vi "main.vi"() -> ()   [LabVIEW 2023] (continued)
8        17\t1F\t08\t60\tB1\t1F\t08\t55\r\n      2944  0CF102A7   00000004    8        30\t75\tE0\t2E\t80\tFF\tFF\tFD\r\n      2943  0C3C4D4A   00000004    8        BE\tFF\tFF\t7F\t18\tFF\tFF\t55\r\n      2943  0CF101A7   00000004    8        68\t00\t97\tCC\t00\t16\t39\tAD\r\n      2942  18F120F0   00000004    8        2B\t75\t60\tB1\tB0\t01\tFF\tFF\r\n      2941  18F11FF0   00000004    8        FF\t3F\t90\t68\t88\t1B\t10\t5C\r\n      2932  1FFFFFFF   00000004    8        00\t00\tFF\tFF\tFF\tFF\tFF\tFF\r\n      2923  0CF102A7   00000004    8        30\t75\tE0\t2E\t80\tFF\tFF\tFD\r\n      2923  0CF101A7   00000004    8        68\t00\t97\tCC\t00\t16\t39\tAC\r\n      2922  1FFFFFFF   00000004    8        00\t20\tFF\tFF\tFF\tFF\tFF\tFF\r\n      2945  18F106A7   00000004    8        00\tF7\tFF\tFF\tFF\tFF\tFF\tAB\r\n      2945  0CF104A7   00000004    8        F0\t60\t22\tFC\tFF\tFF\tFF\t55\r\n      2944  0CF103A7   00000004    8        17\t1F\t08\t60\tB1\t1F\t08\t55\r\n      2944  0CF102A7   00000004    8        30\t75\tE0\t2E\t80\tFF\tFF\tFD\r\n      2943  0C3C4D4A   00000004    8        BE\tFF\tFF\t7F\t18\tFF\tFF\t55\r\n      2943  0CF101A7   00000004    8        68\t00\t97\tCC\t00\t16\t39\tAD\r\n      2942  18F120F0   00000004    8        2B\t75\t60\tB1\tB0\t01\tFF\tFF\r\n      2941  18F11FF0   00000004    8        FF\t3F\t90\t68\t88\t1B\t10\t5C\r\n      2932  1FFFFFFF   00000004    8        00\t00\tFF\tFF\tFF\tFF\tFF\tFF\r\n      2923  0CF102A7   00000004    8        30\t75\tE0\t2E\t80\tFF\tFF\tFD\r\n      2923  0CF101A7   00000004    8        68\t00\t97\tCC\t00\t16\t39\tAC\r\n      2946  18F121F0   00000004    8        09\t19\t00\t00\tFF\tFF\tB0\t01\r\n      2945  18F106A7   00000004    8        00\tF7\tFF\tFF\tFF\tFF\tFF\tAB\r\n      2945  0CF104A7   00000004    8        F0\t60\t22\tFC\tFF\tFF\tFF\t55\r\n      2944  0CF103A7   00000004    8        17\t1F\t08\t60\tB1\t1F\t08\t55\r\n      2944  0CF102A7   00000004    8        30\t75\tE0\t2E\t80\tFF\tFF\tFD\r\n      2943  0C3C4D4A   00000004    8        BE\tFF\tFF\t7F\t18\tFF\tFF\t55\r\n      2943  0CF101A7   00000004    8        68\t00\t97\tCC\t00\t16\t39\tAD\r\n      2942  18F120F0   00000004    8        2B\t75\t60\tB1\tB0\t01\tFF\tFF\r\n      2941  18F11FF0   00000004    8        FF\t3F\t90\t68\t88\t1B\t10\t5C\r\n      2932  1FFFFFFF   00000004    8        00\t00\tFF\tFF\tFF\tFF\tFF\tFF\r\n      2923  0CF102A7   00000004    8        30\t75\tE0\t2E\t80\tFF\tFF\tFD\r\n      2947  1FFFFFFF   00000004    8        00\t20\tFF\tFF\tFF\tFF\tFF\tFF\r\n      2946  18F121F0   00000004    8        09\t19\t00\t00\tFF\tFF\tB0\t01\r\n      2945  18F106A7   00000004    8        00\tF7\tFF\tFF\tFF\tFF\tFF\tAB\r\n      2945  0CF104A7   00000004    8        F0\t60\t22\tFC\tFF\tFF\tFF\t55\r\n      2944  0CF103A7   00000004    8        17\t1F\t08\t60\tB1\t1F\t08\t55\r\n      2944  0CF102A7   00000004    8        30\t75\tE0\t2E\t80\tFF\tFF\tFD\r\n      2943  0C3C4D4A   00000004    8        BE\tFF\tFF\t7F\t18\tFF\tFF\t55\r\n      2943  0CF101A7   00000004    8        68\t00\t97\tCC\t00\t16\t39\tAD\r\n      2942  18F120F0   00000004    8        2B\t75\t60\tB1\tB0\t01\tFF\tFF\r\n      2941  18F11FF0   00000004    8        FF\t3F\t90\t68\t88\t1B\t10\t5C\r\n      2932  1FFFFFFF   00000004    8        00\t00\tFF\tFF\tFF\tFF\tFF\tFF\r\n      2952  1FFFFFFF   00000004    8        00\t20\tFF\tFF\tFF\tFF\tFF\tFF\r\n      2947  1FFFFFFF   00000004    8        00\t20\tFF\tFF\tFF\tFF\tFF\tFF\r\n      2946  18F121F0   00000004    8        09\t19\t00\t00\tFF\tFF\tB0\t01\r\n      2945  18F106A7   00000004    8        00\tF7\tFF\tFF\tFF\tFF\tFF\tAB\r\n      2945  0CF104A7   00000004    8        F0\t60\t22\tFC\tFF\tFF\tFF\t55\r\n      2944  0CF103A7   00000004    8        17\t1F\t08\t60\tB1\t1F\t08\t55\r\n      2944  0CF102A7   00000004    8        30\t75\tE0\t2E\t80\tFF\tFF\tFD\r\n      2943  0C3C4D4A   00000004    8        BE\tFF\tFF\t7F\t18\tFF\tFF\t55\r\n      2943  0CF101A7   00000004    8        68\t00\t97\tCC\t00\t16\t39\tAD\r\n      2942  18F120F0   00000004    8        2B\t75\t60\tB1\tB0\t01\tFF\tFF\r\n      2941  18F11FF0   00000004    8        FF\t3F\t90\t68\t88\t1B\t10\t5C\r\n      2962  1FFFFFFF   00000004    8        00\t20\tFF\tFF\tFF\tFF\tFF\tFF\r\n      2952  1FFFFFFF   00000004    8        00\t20\tFF\tFF\tFF\tFF\tFF\tFF\r\n      2947  1FFFFFFF   00000004    8        00\t20\tFF\tFF\tFF\tFF\tFF\tFF\r\n      2946  18F121F0   00000004    8        09\t19\t00\t00\tFF\tFF\tB0\t01\r\n      2945  18F106A7   00000004    8        00\tF7\tFF\tFF\tFF\tFF\tFF\tAB\r\n      2945  0CF104A7   00000004    8        F0\t60\t22\tFC\tFF\tFF\tFF\t55\r\n      2944  0CF103A7   00000004    8        17\t1F\t08\t60\tB1\t1F\t08\t55\r\n      2944  0CF102A7   00000004    8        30\t75\tE0\t2E\t80\tFF\tFF\tFD\r\n      2943  0C3C4D4A   00000004    8        BE\tFF\tFF\t7F\t18\tFF\tFF\t55\r\n      2943  0CF101A7   00000004    8        68\t00\t97\tCC\t00\t16\t39\tAD\r\n      2942  18F120F0   00000004    8        2B\t75\t60\tB1\tB0\t01\tFF\tFF\r\n      2963  0CF101A7   00000004    8        68\t00\t97\tCC\t00\t16\t39\tAE\r\n      2962  1FFFFFFF   00000004    8        00\t20\tFF\tFF\tFF\tFF\tFF\tFF\r\n      2952  1FFFFFFF   00000004    8        00\t20\tFF\tFF\tFF\tFF\tFF\tFF\r\n      2947  1FFFFFFF   00000004    8        00\t20\tFF\tFF\tFF\tFF\tFF\tFF\r\n      2946  18F121F0   00000004    8        09\t19\t00\t00\tFF\tFF\tB0\t01\r\n      2945  18F106A7   00000004    8        00\tF7\tFF\tFF\tFF\tFF\tFF\tAB\r\n      2945  0CF104A7   00000004    8        F0\t60\t22\tFC\tFF\tFF\tFF\t55\r\n      2944  0CF103A7   00000004    8        17\t1F\t08\t60\tB1\t1F\t08\t55\r\n      2944  0CF102A7   00000004    8        30\t75\tE0\t2E\t80\tFF\tFF\tFD\r\n      2943  0C3C4D4A   00000004    8        BE\tFF\tFF\t7F\t18\tFF\tFF\t55\r\n      2943  0CF101A7   00000004    8        68\t00\t97\tCC\t00\t16\t39\tAD\r\n      2963  0CF102A7   00000004    8        30\t75\tE0\t2E\t80\tFF\tFF\tFD\r\n      2963  0CF101A7   00000004    8        68\t00\t97\tCC\t00\t16\t39\tAE\r\n      2962  1FFFFFFF   00000004    8        00\t20\tFF\tFF\tFF\tFF\tFF\tFF\r\n      2952  1FFFFFFF   00000004    8        00\t20\tFF\tFF\tFF\tFF\tFF\tFF\r\n      2947  1FFFFFFF   00000004    8        00\t20\tFF\tFF\tFF\tFF\tFF\tFF\r\n      2946  18F121F0   00000004    8        09\t19\t00\t00\tFF\tFF\tB0\t01\r\n      2945  18F106A7   00000004    8        00\tF7\tFF\tFF\tFF\tFF\tFF\tAB\r\n      2945  0CF104A7   00000004    8        F0\t60\t22\tFC\tFF\tFF\tFF\t55\r\n      2944  0CF103A7   00000004    8        17\t1F\t08\t60\tB1\t1F\t08\t55\r\n      2944  0CF102A7   00000004    8        30\t75\tE0\t2E\t80\tFF\tFF\tFD\r\n      2943  0C3C4D4A   00000004    8        BE\tFF\tFF\t7F\t18\tFF\tFF\t55\r\n      2972  1FFFFFFF   00000004    8        00\t20\tFF\tFF\tFF\tFF\tFF\tFF\r\n      2963  0CF102A7   00000004    8        30\t75\tE0\t2E\t80\tFF\tFF\tFD\r\n      2963  0CF101A7   00000004    8        68\t00\t97\tCC\t00\t16\t39\tAE\r\n      2962  1FFFFFFF   00000004    8        00\t20\tFF\tFF\tFF\tFF\tFF\tFF\r\n      2952  1FFFFFFF   00000004    8        00\t20\tFF\tFF\tFF\tFF\tFF\tFF\r\n      2947  1FFFFFFF   00000004    8        00\t20\tFF\tFF\tFF\tFF\tFF\tFF\r\n      2946  18F121F0   00000004    8        09\t19\t00\t00\tFF\tFF\tB0\t01\r\n      2945  18F106A7   00000004    8        00\tF7\tFF\tFF\tFF\tFF\tFF\tAB\r\n      2945  0CF104A7   00000004    8        F0\t60\t22\tFC\tFF\tFF\tFF\t55\r\n      2944  0CF103A7   00000004    8        17\t1F\t08\t60\tB1\t1F\t08\t55\r\n      2944  0CF102A7   00000004    8        30\t75\tE0\t2E\t80\tFF\tFF\tFD\r\n      2982  1FFFFFFF   00000004    8        00\t00\tFF\tFF\tFF\tFF\tFF\tFF\r\n      2972  1FFFFFFF   00000004    8        00\t20\tFF\tFF\tFF\tFF\tFF\tFF\r\n      2963  0CF102A7   00000004    8        30\t75\tE0\t2E\t80\tFF\tFF\tFD\r\n      2963  0CF101A7   00000004    8        68\t00\t97\tCC\t00\t16\t39\tAE\r\n      2962  1FFFFFFF   00000004    8        00\t20\tFF\tFF\tFF\tFF\tFF\tFF\r\n      2952  1FFFFFFF   00000004    8        00\t20\tFF\tFF\tFF\tFF\tFF\tFF\r\n      2947  1FFFFFFF   00000004    8        00\t20\tFF\tFF\tFF\tFF\tFF\tFF\r\n      2946  18F121F0   00000004    8        09\t19\t00\t00\tFF\tFF\tB0\t01\r\n      2945  18F106A7   00000004    8        00\tF7\tFF\tFF\tFF\tFF\tFF\tAB\r\n      2945  0CF104A7   00000004    8        F0\t60\t22\tFC\tFF\tFF\tFF\t55\r\n      2944  0CF103A7   00000004    8        17\t1F\t08\t60\tB1\t1F\t08\t55\r\n      2983  0CF101A7   00000004    8        68\t00\t97\tCC\t00\t16\t39\tAF\r\n      2982  1FFFFFFF   00000004    8        00\t00\tFF\tFF\tFF\tFF\tFF\tFF\r\n      2972  1FFFFFFF   00000004    8        00\t20\tFF\tFF\tFF\tFF\tFF\tFF\r\n      2963  0CF102A7   00000004    8        30\t75\tE0\t2E\t80\tFF\tFF\tFD\r\n      2963  0CF101A7   00000004    8        68\t00\t97\tCC\t00\t16\t39\tAE\r\n      2962  1FFFFFFF   00000004    8        00\t20\tFF\tFF\tFF\tFF\tFF\tFF\r\n      2952  1FFFFFFF   00000004    8        00\t20\tFF\tFF\tFF\tFF\tFF\tFF\r\n      2947  1FFFFFFF   00000004    8        00\t20\tFF\tFF\tFF\tFF\tFF\tFF\r\n      2946  18F121F0   00000004    8        09\t19\t00\t00\tFF\tFF\tB0\t01\r\n      2945  18F106A7   00000004    8        00\tF7\tFF\tFF\tFF\tFF\tFF\tAB\r\n      2945  0CF104A7   00000004    8        F0\t60\t22\tFC\tFF\tFF\tFF\t55\r\n      2983  0CF102A7   00000004    8        30\t75\tE0\t2E\t80\tFF\tFF\tFD\r\n      2983  0CF101A7   00000004    8        68\t00\t97\tCC\t00\t16\t39\tAF\r\n      2982  1FFFFFFF   00000004    8        00\t00\tFF\tFF\tFF\tFF\tFF\tFF\r\n      2972  1FFFFFFF   00000004    8        00\t20\tFF\tFF\tFF\tFF\tFF\tFF\r\n      2963  0CF102A7   00000004    8        30\t75\tE0\t2E\t80\tFF\tFF\tFD\r\n      2963  0CF101A7   00000004    8        68\t00\t97\tCC\t00\t16\t39\tAE\r\n      2962  1FFFFFFF   00000004    8        00\t20\tFF\tFF\tFF\tFF\tFF\tFF\r\n      2952  1FFFFFFF   00000004    8        00\t20\tFF\tFF\tFF\tFF\tFF\tFF\r\n      2947  1FFFFFFF   00000004    8        00\t20\tFF\tFF\tFF\tFF\tFF\tFF\r\n      2946  18F121F0   00000004    8        09\t19\t00\t00\tFF\tFF\tB0\t01\r\n      2945  18F106A7   00000004    8        00\tF7\tFF\tFF\tFF\tFF\tFF\tAB\r\n      2992  1FFFFFFF   00000004    8        00\t20\tFF\tFF\tFF\tFF\tFF\tFF\r\n      2983  0CF102A7   00000004    8        30\t75\tE0\t2E\t80\tFF\tFF\tFD\r\n      2983  0CF101A7   00000004    8        68\t00\t97\tCC\t00\t16\t39\tAF\r\n      2982  1FFFFFFF   00000004    8        00\t00\tFF\tFF\tFF\tFF\tFF\tFF\r\n      2972  1FFFFFFF   00000004    8        00\t20\tFF\tFF\tFF\tFF\tFF\tFF\r\n      2963  0CF102A7   00000004    8        30\t75\tE0\t2E\t80\tFF\tFF\tFD\r\n      2963  0CF101A7   00000004    8        68\t00\t97\tCC\t00\t16\t39\tAE\r\n      2962  1FFFFFFF   00000004    8        00\t20\tFF\tFF\tFF\tFF\tFF\tFF\r\n      2952  1FFFFFFF   00000004    8        00\t20\tFF\tFF\tFF\tFF\tFF\tFF\r\n      2947  1FFFFFFF   00000004    8        00\t20\tFF\tFF\tFF\tFF\tFF\tFF\r\n      2946  18F121F0   00000004    8        09\t19\t00\t00\tFF\tFF\tB0\t01\r\n      2993  18F106A7   00000004    8        00\tF7\tFF\tFF\tFF\tFF\tFF\tAC\r\n      2992  1FFFFFFF   00000004    8        00\t20\tFF\tFF\tFF\tFF\tFF\tFF\r\n      2983  0CF102A7   00000004    8        30\t75\tE0\t2E\t80\tFF\tFF\tFD\r\n      2983  0CF101A7   00000004    8        68\t00\t97\tCC\t00\t16\t39\tAF\r\n      2982  1FFFFFFF   00000004    8        00\t00\tFF\tFF\tFF\tFF\tFF\tFF\r\n      2972  1FFFFFFF   00000004    8        00\t20\tFF\tFF\tFF\tFF\tFF\tFF\r\n      2963  0CF102A7   00000004    8        30\t75\tE0\t2E\t80\tFF\tFF\tFD\r\n      2963  0CF101A7   00000004    8        68\t00\t97\tCC\t00\t16\t39\tAE\r\n      2962  1FFFFFFF   00000004    8        00\t20\tFF\tFF\tFF\tFF\tFF\tFF\r\n      2952  1FFFFFFF   00000004    8        00\t20\tFF\tFF\tFF\tFF\tFF\tFF\r\n      2947  1FFFFFFF   00000004    8        00\t20\tFF\tFF\tFF\tFF\tFF\tFF\r\n      3002  1FFFFFFF   00000004    8        00\t00\tFF\tFF\tFF\tFF\tFF\tFF\r\n      2993  18F106A7   00000004    8        00\tF7\tFF\tFF\tFF\tFF\tFF\tAC\r\n      2992  1FFFFFFF   00000004    8        00\t20\tFF\tFF\tFF\tFF\tFF\tFF\r\n      2983  0CF102A7   00000004    8        30\t75\tE0\t2E\t80\tFF\tFF\tFD\r\n      2983  0CF101A7   00000004    8        68\t00\t97\tCC\t00\t16\t39\tAF\r\n      2982  1FFFFFFF   00000004    8        00\t00\tFF\tFF\tFF\tFF\tFF\tFF\r\n      2972  1FFFFFFF   00000004    8        00\t20\tFF\tFF\tFF\tFF\tFF\tFF\r\n      2963  0CF102A7   00000004    8        30\t75\tE0\t2E\t80\tFF\tFF\tFD\r\n      2963  0CF101A7   00000004    8        68\t00\t97\tCC\t00\t16\t39\tAE\r\n      2962  1FFFFFFF   00000004    8        00\t20\tFF\tFF\tFF\tFF\tFF\tFF\r\n      2952  1FFFFFFF   00000004    8        00\t20\tFF\tFF\tFF\tFF\tFF\tFF\r\n      3003  0CF101A7   00000004    8        68\t00\t97\tCC\t00\t16\t39\tB0\r\n      3002  1FFFFFFF   00000004    8        00\t00\tFF\tFF\tFF\tFF\tFF\tFF\r\n      2993  18F106A7   00000004    8        00\tF7\tFF\tFF\tFF\tFF\tFF\tAC\r\n      2992  1FFFFFFF   00000004    8        00\t20\tFF\tFF\tFF\tFF\tFF\tFF\r\n      2983  0CF102A7   00000004    8        30\t75\tE0\t2E\t80\tFF\tFF\tFD\r\n      2983  0CF101A7   00000004    8        68\t00\t97\tCC\t00\t16\t39\tAF\r\n      2982  1FFFFFFF   00000004    8        00\t00\tFF\tFF\tFF\tFF\tFF\tFF\r\n      2972  1FFFFFFF   00000004    8        00\t20\tFF\tFF\tFF\tFF\tFF\tFF\r\n      2963  0CF102A7   00000004    8        30\t75\tE0\t2E\t80\tFF\tFF\tFD\r\n      2963  0CF101A7   00000004    8        68\t00\t97\tCC\t00\t16\t39\tAE\r\n      2962  1FFFFFFF   00000004    8        00\t20\tFF\tFF\tFF\tFF\tFF\tFF\r\n      3003  0CF102A7   00000004    8        30\t75\tE0\t2E\t80\tFF\tFF\tFD\r\n      3003  0CF101A7   00000004    8        68\t00\t97\tCC\t00\t16\t39\tB0\r\n      3002  1FFFFFFF   00000004    8        00\t00\tFF\tFF\tFF\tFF\tFF\tFF\r\n      2993  18F106A7   00000004    8        00\tF7\tFF\tFF\tFF\tFF\tFF\tAC\r\n      2992  1FFFFFFF   00000004    8        00\t20\tFF\tFF\tFF\tFF\tFF\tFF\r\n      2983  0CF102A7   00000004    8        30\t75\tE0\t2E\t80\tFF\tFF\tFD\r\n      2983  0CF101A7   00000004    8        68\t00\t97\tCC\t00\t16\t39\tAF\r\n      2982  1FFFFFFF   00000004    8        00\t00\tFF\tFF\tFF\tFF\tFF\tFF\r\n      2972  1FFFFFFF   00000004    8        00\t20\tFF\tFF\tFF\tFF\tFF\tFF\r\n      2963  0CF102A7   00000004    8        30\t75\tE0\t2E\t80\tFF\tFF\tFD\r\n      2963  0CF101A7   00000004    8        68\t00\t97\tCC\t00\t16\t39\tAE\r\n      3012  1FFFFFFF   00000004    8        00\t20\tFF\tFF\tFF\tFF\tFF\tFF\r\n      3003  0CF102A7   00000004    8        30\t75\tE0\t2E\t80\tFF\tFF\tFD\r\n      3003  0CF101A7   00000004    8        68\t00\t97\tCC\t00\t16\t39\tB0\r\n      3002  1FFFFFFF   00000004    8        00\t00\tFF\tFF\tFF\tFF\tFF\tFF\r\n      2993  18F106A7   00000004    8        00\tF7\tFF\tFF\tFF\tFF\tFF\tAC\r\n      2992  1FFFFFFF   00000004    8        00\t20\tFF\tFF\tFF\tFF\tFF\tFF\r\n      2983  0CF102A7   00000004    8        30\t75\tE0\t2E\t80\tFF\tFF\tFD\r\n      2983  0CF101A7   00000004    8        68\t00\t97\tCC\t00\t16\t39\tAF\r\n      2982  1FFFFFFF   00000004    8        00\t00\tFF\tFF\tFF\tFF\tFF\tFF\r\n      2972  1FFFFFFF   00000004    8        00\t20\tFF\tFF\tFF\tFF\tFF\tFF\r\n      2963  0CF102A7   00000004    8        30\t75\tE0\t2E\t80\tFF\tFF\tFD\r\n      3022  1FFFFFFF   00000004    8        00\t00\tFF\tFF\tFF\tFF\tFF\tFF\r\n      3012  1FFFFFFF   00000004    8        00\t20\tFF\tFF\tFF\tFF\tFF\tFF\r\n      3003  0CF102A7   00000004    8        30\t75\tE0\t2E\t80\tFF\tFF\tFD\r\n      3003  0CF101A7   00000004    8        68\t00\t97\tCC\t00\t16\t39\tB0\r\n      3002  1FFFFFFF   00000004    8        00\t00\tFF\tFF\tFF\tFF\tFF\tFF\r\n      2993  18F106A7   00000004    8        00\tF7\tFF\tFF\tFF\tFF\tFF\tAC\r\n      2992  1FFFFFFF   00000004    8        00\t20\tFF\tFF\tFF\tFF\tFF\tFF\r\n      2983  0CF102A7   00000004    8        30\t75\tE0\t2E\t80\tFF\tFF\tFD\r\n      2983  0CF101A7   00000004    8        68\t00\t97\tCC\t00\t16\t39\tAF\r\n      2982  1FFFFFFF   00000004    8        00\t00\tFF\tFF\tFF\tFF\tFF\tFF\r\n      2972  1FFFFFFF   00000004    8        00\t20\tFF\tFF\tFF\tFF\tFF\tFF\r\n      3023  0CF101A7   00000004    8        68\t00\t97\tCC\t00\t16\t39\tB1\r\n      3022  1FFFFFFF   00000004    8        00\t00\tFF\tFF\tFF\tFF\tFF\tFF\r\n      3012  1FFFFFFF   00000004    8        00\t20\tFF\tFF\tFF\tFF\tFF\tFF\r\n      3003  0CF102A7   00000004    8        30\t75\tE0\t2E\t80\tFF\tFF\tFD\r\n      3003  0CF101A7   00000004    8        68\t00\t97\tCC\t00\t16\t39\tB0\r\n      3002  1FFFFFFF   00000004    8        00\t00\tFF\tFF\tFF\tFF\tFF\tFF\r\n      2993  18F106A7   00000004    8        00\tF7\tFF\tFF\tFF\tFF\tFF\tAC\r\n      2992  1FFFFFFF   00000004    8        00\t20\tFF\tFF\tFF\tFF\tFF\tFF\r\n      2983  0CF102A7   00000004    8        30\t75\tE0\t2E\t80\tFF\tFF\tFD\r\n      2983  0CF101A7   00000004    8        68\t00\t97\tCC\t00\t16\t39\tAF\r\n      2982  1FFFFFFF   00000004    8        00\t00\tFF\tFF\tFF\tFF\tFF\tFF\r\n      3023  0CF102A7   00000004    8        30\t75\tE0\t2E\t80\tFF\tFF\tFD\r\n      3023  0CF101A7   00000004    8        68\t00\t97\tCC\t00\t16\t39\tB1\r\n      3022  1FFFFFFF   00000004    8        00\t00\tFF\tFF\tFF\tFF\tFF\tFF\r\n      3012  1FFFFFFF   00000004    8        00\t20\tFF\tFF\tFF\tFF\tFF\tFF\r\n      3003  0CF102A7   00000004    8        30\t75\tE0\t2E\t80\tFF\tFF\tFD\r\n      3003  0CF101A7   00000004    8        68\t00\t97\tCC\t00\t16\t39\tB0\r\n      3002  1FFFFFFF   00000004    8        00\t00\tFF\tFF\tFF\tFF\tFF\tFF\r\n      2993  18F106A7   00000004    8        00\tF7\tFF\tFF\tFF\tFF\tFF\tAC\r\n      2992  1FFFFFFF   00000004    8        00\t20\tFF\tFF\tFF\tFF\tFF\tFF\r\n      2983  0CF102A7   00000004    8        30\t75\tE0\t2E\t80\tFF\tFF\tFD\r\n      2983  0CF101A7   00000004    8        68\t00\t97\tCC\t00\t16\t39\tAF\r\n      3032  1FFFFFFF   00000004    8        00\t20\tFF\tFF\tFF\tFF\tFF\tFF\r\n      3023  0CF102A7   00000004    8        30\t75\tE0\t2E\t80\tFF\tFF\tFD\r\n      3023  0CF101A7   00000004    8        68\t00\t97\tCC\t00\t16\t39\tB1\r\n      3022  1FFFFFFF   00000004    8        00\t00\tFF\tFF\tFF\tFF\tFF\tFF\r\n      3012  1FFFFFFF   00000004    8        00\t20\tFF\tFF\tFF\tFF\tFF\tFF\r\n      3003  0CF102A7   00000004    8        30\t75\tE0\t2E\t80\tFF\tFF\tFD\r\n      3003  0CF101A7   00000004    8        68\t00\t97\tCC\t00\t16\t39\tB0\r\n      3002  1FFFFFFF   00000004    8        00\t00\tFF\tFF\tFF\tFF\tFF\tFF\r\n      2993  18F106A7   00000004    8        00\tF7\tFF\tFF\tFF\tFF\tFF\tAC\r\n      2992  1FFFFFFF   00000004    8        00\t20\tFF\tFF\tFF\tFF\tFF\tFF\r\n      2983  0CF102A7   00000004    8        30\t75\tE0\t2E\t80\tFF\tFF\tFD\r\n      3041  18F11FF0   00000004    8        FF\t3F\t90\t68\t88\t1B\t10\t6C\r\n      3032  1FFFFFFF   00000004    8        00\t20\tFF\tFF\tFF\tFF\tFF\tFF\r\n      3023  0CF102A7   00000004    8        30\t75\tE0\t2E\t80\tFF\tFF\tFD\r\n      3023  0CF101A7   00000004    8        68\t00\t97\tCC\t00\t16\t39\tB1\r\n      3022  1FFFFFFF   00000004    8        00\t00\tFF\tFF\tFF\tFF\tFF\tFF\r\n      3012  1FFFFFFF   00000004    8        00\t20\tFF\tFF\tFF\tFF\tFF\tFF\r\n      3003  0CF102A7   00000004    8        30\t75\tE0\t2E\t80\tFF\tFF\tFD\r\n      3003  0CF101A7   00000004    8        68\t00\t97\tCC\t00\t16\t39\tB0\r\n      3002  1FFFFFFF   00000004    8        00\t00\tFF\tFF\tFF\tFF\tFF\tFF\r\n      2993  18F106A7   00000004    8        00\tF7\tFF\tFF\tFF\tFF\tFF\tAC\r\n      2992  1FFFFFFF   00000004    8        00\t20\tFF\tFF\tFF\tFF\tFF\tFF\r\n      3042  18F120F0   00000004    8        2B\t75\t60\tB1\tB0\t01\tFF\tFF\r\n      3041  18F11FF0   00000004    8        FF\t3F\t90\t68\t88\t1B\t10\t6C\r\n      3032  1FFFFFFF   00000004    8        00\t20\tFF\tFF\tFF\tFF\tFF\tFF\r\n      3023  0CF102A7   00000004    8        30\t75\tE0\t2E\t80\tFF\tFF\tFD\r\n      3023  0CF101A7   00000004    8        68\t00\t97\tCC\t00\t16\t39\tB1\r\n      3022  1FFFFFFF   00000004    8        00\t00\tFF\tFF\tFF\tFF\tFF\tFF\r\n      3012  1FFFFFFF   00000004    8        00\t20\tFF\tFF\tFF\tFF\tFF\tFF\r\n      3003  0CF102A7   00000004    8        30\t75\tE0\t2E\t80\tFF\tFF\tFD\r\n      3003  0CF101A7   00000004    8        68\t00\t97\tCC\t00\t16\t39\tB0\r\n      3002  1FFFFFFF   00000004    8        00\t00\tFF\tFF\tFF\tFF\tFF\tFF\r\n      2993  18F106A7   00000004    8        00\tF7\tFF\tFF\tFF\tFF\tFF\tAC\r\n      3043  0CF101A7   00000004    8        68\t00\t97\tCC\t00\t16\t39\tB2\r\n      3042  18F120F0   00000004    8        2B\t75\t60\tB1\tB0\t01\tFF\tFF\r\n      3041  18F11FF0   00000004    8        FF\t3F\t90\t68\t88\t1B\t10\t6C\r\n      3032  1FFFFFFF   00000004    8        00\t20\tFF\tFF\tFF\tFF\tFF\tFF\r\n      3023  0CF102A7   00000004    8        30\t75\tE0\t2E\t80\tFF\tFF\tFD\r\n      3023  0CF101A7   00000004    8        68\t00\t97\tCC\t00\t16\t39\tB1\r\n      3022  1FFFFFFF   00000004    8        00\t00\tFF\tFF\tFF\tFF\tFF\tFF\r\n      3012  1FFFFFFF   00000004    8        00\t20\tFF\tFF\tFF\tFF\tFF\tFF\r\n      3003  0CF102A7   00000004    8        30\t75\tE0\t2E\t80\tFF\tFF\tFD\r\n      3003  0CF101A7   00000004    8        68\t00\t97\tCC\t00\t16\t39\tB0\r\n      3002  1FFFFFFF   00000004    8        00\t00\tFF\tFF\tFF\tFF\tFF\tFF\r\n      3043  0C3C4D4A   00000004    8        BE\tFF\tFF\t7F\t18\tFF\tFF\t56\r\n      3043  0CF101A7   00000004    8        68\t00\t97\tCC\t00\t16\t39\tB2\r\n      3042  18F120F0   00000004    8        2B\t75\t60\tB1\tB0\t01\tFF\tFF\r\n      3041  18F11FF0   00000004    8        FF\t3F\t90\t68\t88\t1B\t10\t6C\r\n      3032  1FFFFFFF   00000004    8        00\t20\tFF\tFF\tFF\tFF\tFF\tFF\r\n      3023  0CF102A7   00000004    8        30\t75\tE0\t2E\t80\tFF\tFF\tFD\r\n      3023  0CF101A7   00000004    8        68\t00\t97\tCC\t00\t16\t39\tB1\r\n      3022  1FFFFFFF   00000004    8        00\t00\tFF\tFF\tFF\tFF\tFF\tFF\r\n      3012  1FFFFFFF   00000004    8        00\t20\tFF\tFF\tFF\tFF\tFF\tFF\r\n      3003  0CF102A7   00000004    8        30\t75\tE0\t2E\t80\tFF\tFF\tFD\r\n      3003  0CF101A7   00000004    8        68\t00\t97\tCC\t00\t16\t39\tB0\r\n      3044  0CF102A7   00000004    8        30\t75\tE0\t2E\t80\tFF\tFF\tFD\r\n      3043  0C3C4D4A   00000004    8        BE\tFF\tFF\t7F\t18\tFF\tFF\t56\r\n      3043  0CF101A7   00000004    8        68\t00\t97\tCC\t00\t16\t39\tB2\r\n      3042  18F120F0   00000004    8        2B\t75\t60\tB1\tB0\t01\tFF\tFF\r\n      3041  18F11FF0   00000004    8        FF\t3F\t90\t68\t88\t1B\t10\t6C\r\n      3032  1FFFFFFF   00000004    8        00\t20\tFF\tFF\tFF\tFF\tFF\tFF\r\n      3023  0CF102A7   00000004    8        30\t75\tE0\t2E\t80\tFF\tFF\tFD\r\n      3023  0CF101A7   00000004    8        68\t00\t97\tCC\t00\t16\t39\tB1\r\n      3022  1FFFFFFF   00000004    8        00\t00\tFF\tFF\tFF\tFF\tFF\tFF\r\n      3012  1FFFFFFF   00000004    8        00\t20\tFF\tFF\tFF\tFF\tFF\tFF\r\n      3003  0CF102A7   00000004    8        30\t75\tE0\t2E\t80\tFF\tFF\tFD\r\n      3044  0CF103A7   00000004    8        17\t1F\t08\t60\tB1\t1F\t08\t56\r\n      3044  0CF102A7   00000004    8        30\t75\tE0\t2E\t80\tFF\tFF\tFD\r\n      3043  0C3C4D4A   00000004    8        BE\tFF\tFF\t7F\t18\tFF\tFF\t56\r\n      3043  0CF101A7   00000004    8        68\t00\t97\tCC\t00\t16\t39\tB2\r\n      3042  18F120F0   00000004    8        2B\t75\t60\tB1\tB0\t01\tFF\tFF\r\n      3041  18F11FF0   00000004    8        FF\t3F\t90\t68\t88\t1B\t10\t6C\r\n      3032  1FFFFFFF   00000004    8        00\t20\tFF\tFF\tFF\tFF\tFF\tFF\r\n      3023  0CF102A7   00000004    8        30\t75\tE0\t2E\t80\tFF\tFF\tFD\r\n      3023  0CF101A7   00000004    8        68\t00\t97\tCC\t00\t16\t39\tB1\r\n      3022  1FFFFFFF   00000004    8        00\t00\tFF\tFF\tFF\tFF\tFF\tFF\r\n      3012  1FFFFFFF   00000004    8        00\t20\tFF\tFF\tFF\tFF\tFF\tFF\r\n      3045  0CF104A7   00000004    8        F0\t60\t22\tFC\tFF\tFF\tFF\t56\r\n      3044  0CF103A7   00000004    8        17\t1F\t08\t60\tB1\t1F\t08\t56\r\n      3044  0CF102A7   00000004    8        30\t75\tE0\t2E\t80\tFF\tFF\tFD\r\n      3043  0C3C4D4A   00000004    8        BE\tFF\tFF\t7F\t18\tFF\tFF\t56\r\n      3043  0CF101A7   00000004    8        68\t00\t97\tCC\t00\t16\t39\tB2\r\n      3042  18F120F0   00000004    8        2B\t75\t60\tB1\tB0\t01\tFF\tFF\r\n      3041  18F11FF0   00000004    8        FF\t3F\t90\t68\t88\t1B\t10\t6C\r\n      3032  1FFFFFFF   00000004    8        00\t20\tFF\tFF\tFF\tFF\tFF\tFF\r\n      3023  0CF102A7   00000004    8        30\t75\tE0\t2E\t80\tFF\tFF\tFD\r\n      3023  0CF101A7   00000004    8        68\t00\t97\tCC\t00\t16\t39\tB1\r\n      3022  1FFFFFFF   00000004    8        00\t00\tFF\tFF\tFF\tFF\tFF\tFF\r\n      3045  18F106A7   00000004    8        00\tF7\tFF\tFF\tFF\tFF\tFF\tAD\r\n      3045  0CF104A7   00000004    8        F0\t60\t22\tFC\tFF\tFF\tFF\t56\r\n      3044  0CF103A7   00000004    8        17\t1F\t08\t60\tB1\t1F\t08\t56\r\n      3044  0CF102A7   00000004    8        30\t75\tE0\t2E\t80\tFF\tFF\tFD\r\n      3043  0C3C4D4A   00000004    8        BE\tFF\tFF\t7F\t18\tFF\tFF\t56\r\n      3043  0CF101A7   00000004    8        68\t00\t97\tCC\t00\t16\t39\tB2\r\n      3042  18F120F0   00000004    8        2B\t75\t60\tB1\tB0\t01\tFF\tFF\r\n      3041  18F11FF0   00000004    8        FF\t3F\t90\t68\t88\t1B\t10\t6C\r\n      3032  1FFFFFFF   00000004    8        00\t20\tFF\tFF\tFF\tFF\tFF\tFF\r\n      3023  0CF102A7   00000004    8        30\t75\tE0\t2E\t80\tFF\tFF\tFD\r\n      3023  0CF101A7   00000004    8        68\t00\t97\tCC\t00\t16\t39\tB1\r\n      3046  18F121F0   00000004    8        09\t33\t00\t00\tFF\tFF\tB0\t01\r\n      3045  18F106A7   00000004    8        00\tF7\tFF\tFF\tFF\tFF\tFF\tAD\r\n      3045  0CF104A7   00000004    8        F0\t60\t22\tFC\tFF\tFF\tFF\t56\r\n      3044  0CF103A7   00000004    8        17\t1F\t08\t60\tB1\t1F\t08\t56\r\n      3044  0CF102A7   00000004    8        30\t75\tE0\t2E\t80\tFF\tFF\tFD\r\n      3043  0C3C4D4A   00000004    8        BE\tFF\tFF\t7F\t18\tFF\tFF\t56\r\n      3043  0CF101A7   00000004    8        68\t00\t97\tCC\t00\t16\t39\tB2\r\n      3042  18F120F0   00000004    8        2B\t75\t60\tB1\tB0\t01\tFF\tFF\r\n      3041  18F11FF0   00000004    8        FF\t3F\t90\t68\t88\t1B\t10\t6C\r\n      3032  1FFFFFFF   00000004    8        00\t20\tFF\tFF\tFF\tFF\tFF\tFF\r\n      3023  0CF102A7   00000004    8        30\t75\tE0\t2E\t80\tFF\tFF\tFD\r\n      3047  1FFFFFFF   00000004    8        00\t20\tFF\tFF\tFF\tFF\tFF\tFF\r\n      3046  18F121F0   00000004    8        09\t33\t00\t00\tFF\tFF\tB0\t01\r\n      3045  18F106A7   00000004    8        00\tF7\tFF\tFF\tFF\tFF\tFF\tAD\r\n      3045  0CF104A7   00000004    8        F0\t60\t22\tFC\tFF\tFF\tFF\t56\r\n      3044  0CF103A7   00000004    8        17\t1F\t08\t60\tB1\t1F\t08\t56\r\n      3044  0CF102A7   00000004    8        30\t75\tE0\t2E\t80\tFF\tFF\tFD\r\n      3043  0C3C4D4A   00000004    8        BE\tFF\tFF\t7F\t18\tFF\tFF\t56\r\n      3043  0CF101A7   00000004    8        68\t00\t97\tCC\t00\t16\t39\tB2\r\n      3042  18F120F0   00000004    8        2B\t75\t60\tB1\tB0\t01\tFF\tFF\r\n      3041  18F11FF0   00000004    8        FF\t3F\t90\t68\t88\t1B\t10\t6C\r\n      3032  1FFFFFFF   00000004    8        00\t20\tFF\tFF\tFF\tFF\tFF\tFF\r\n      3052  1FFFFFFF   00000004    8        00\t20\tFF\tFF\tFF\tFF\tFF\tFF\r\n      3047  1FFFFFFF   00000004    8        00\t20\tFF\tFF\tFF\tFF\tFF\tFF\r\n      3046  18F121F0   00000004    8        09\t33\t00\t00\tFF\tFF\tB0\t01\r\n      3045  18F106A7   00000004    8        00\tF7\tFF\tFF\tFF\tFF\tFF\tAD\r\n      3045  0CF104A7   00000004    8        F0\t60\t22\tFC\tFF\tFF\tFF\t56\r\n      3044  0CF103A7   00000004    8        17\t1F\t08\t60\tB1\t1F\t08\t56\r\n      3044  0CF102A7   00000004    8        30\t75\tE0\t2E\t80\tFF\tFF\tFD\r\n      3043  0C3C4D4A   00000004    8        BE\tFF\tFF\t7F\t18\tFF\tFF\t56\r\n      3043  0CF101A7   00000004    8        68\t00\t97\tCC\t00\t16\t39\tB2\r\n      3042  18F120F0   00000004    8        2B\t75\t60\tB1\tB0\t01\tFF\tFF\r\n      3041  18F11FF0   00000004    8        FF\t3F\t90\t68\t88\t1B\t10\t6C\r\n      3062  1FFFFFFF   00000004    8        00\t20\tFF\tFF\tFF\tFF\tFF\tFF\r\n      3052  1FFFFFFF   00000004    8        00\t20\tFF\tFF\tFF\tFF\tFF\tFF\r\n      3047  1FFFFFFF   00000004    8        00\t20\tFF\tFF\tFF\tFF\tFF\tFF\r\n      3046  18F121F0   00000004    8        09\t33\t00\t00\tFF\tFF\tB0\t01\r\n      3045  18F106A7   00000004    8        00\tF7\tFF\tFF\tFF\tFF\tFF\tAD\r\n      3045  0CF104A7   00000004    8        F0\t60\t22\tFC\tFF\tFF\tFF\t56\r\n      3044  0CF103A7   00000004    8        17\t1F\t08\t60\tB1\t1F\t08\t56\r\n      3044  0CF102A7   00000004    8        30\t75\tE0\t2E\t80\tFF\tFF\tFD\r\n      3043  0C3C4D4A   00000004    8        BE\tFF\tFF\t7F\t18\tFF\tFF\t56\r\n      3043  0CF101A7   00000004    8        68\t00\t97\tCC\t00\t16\t39\tB2\r\n      3042  18F120F0   00000004    8        2B\t75\t60\tB1\tB0\t01\tFF\tFF\r\n      3063  0CF101A7   00000004    8        68\t00\t97\tCC\t00\t16\t39\tB3\r\n      3062  1FFFFFFF   00000004    8        00\t20\tFF\tFF\tFF\tFF\tFF\tFF\r\n      3052  1FFFFFFF   00000004    8        00\t20\tFF\tFF\tFF\tFF\tFF\tFF\r\n      3047  1FFFFFFF   00000004    8        00\t20\tFF\tFF\tFF\tFF\tFF\tFF\r\n      3046  18F121F0   00000004    8        09\t33\t00\t00\tFF\tFF\tB0\t01\r\n      3045  18F106A7   00000004    8        00\tF7\tFF\tFF\tFF\tFF\tFF\tAD\r\n      3045  0CF104A7   00000004    8        F0\t60\t22\tFC\tFF\tFF\tFF\t56\r\n      3044  0CF103A7   00000004    8        17\t1F\t08\t60\tB1\t1F\t08\t56\r\n      3044  0CF102A7   00000004    8        30\t75\tE0\t2E\t80\tFF\tFF\tFD\r\n      3043  0C3C4D4A   00000004    8        BE\tFF\tFF\t7F\t18\tFF\tFF\t56\r\n      3043  0CF101A7   00000004    8        68\t00\t97\tCC\t00\t16\t39\tB2\r\n      3063  0CF102A7   00000004    8        30\t75\tE0\t2E\t80\tFF\tFF\tFD\r\n      3063  0CF101A7   00000004    8        68\t00\t97\tCC\t00\t16\t39\tB3\r\n      3062  1FFFFFFF   00000004    8        00\t20\tFF\tFF\tFF\tFF\tFF\tFF\r\n      3052  1FFFFFFF   00000004    8        00\t20\tFF\tFF\tFF\tFF\tFF\tFF\r\n      3047  1FFFFFFF   00000004    8        00\t20\tFF\tFF\tFF\tFF\tFF\tFF\r\n      3046  18F121F0   00000004    8        09\t33\t00\t00\tFF\tFF\tB0\t01\r\n      3045  18F106A7   00000004    8        00\tF7\tFF\tFF\tFF\tFF\tFF\tAD\r\n      3045  0CF104A7   00000004    8        F0\t60\t22\tFC\tFF\tFF\tFF\t56\r\n      3044  0CF103A7   00000004    8        17\t1F\t08\t60\tB1\t1F\t08\t56\r\n      3044  0CF102A7   00000004    8        30\t75\tE0\t2E\t80\tFF\tFF\tFD\r\n      3043  0C3C4D4A   00000004    8        BE\tFF\tFF\t7F\t18\tFF\tFF\t56\r\n      3072  1FFFFFFF   00000004    8        00\t20\tFF\tFF\tFF\tFF\tFF\tFF\r\n      3063  0CF102A7   00000004    8        30\t75\tE0\t2E\t80\tFF\tFF\tFD\r\n      3063  0CF101A7   00000004    8        68\t00\t97\tCC\t00\t16\t39\tB3\r\n      3062  1FFFFFFF   00000004    8        00\t20\tFF\tFF\tFF\tFF\tFF\tFF\r\n      3052  1FFFFFFF   00000004    8        00\t20\tFF\tFF\tFF\tFF\tFF\tFF\r\n      3047  1FFFFFFF   00000004    8        00\t20\tFF\tFF\tFF\tFF\tFF\tFF\r\n      3046  18F121F0   00000004    8        09\t33\t00\t00\tFF\tFF\tB0\t01\r\n      3045  18F106A7   00000004    8        00\tF7\tFF\tFF\tFF\tFF\tFF\tAD\r\n      3045  0CF104A7   00000004    8        F0\t60\t22\tFC\tFF\tFF\tFF\t56\r\n      3044  0CF103A7   00000004    8        17\t1F\t08\t60\tB1\t1F\t08\t56\r\n      3044  0CF102A7   00000004    8        30\t75\tE0\t2E\t80\tFF\tFF\tFD\r\n      3082  1FFFFFFF   00000004    8        00\t20\tFF\tFF\tFF\tFF\tFF\tFF\r\n      3072  1FFFFFFF   00000004    8        00\t20\tFF\tFF\tFF\tFF\tFF\tFF\r\n      3063  0CF102A7   00000004    8        30\t75\tE0\t2E\t80\tFF\tFF\tFD\r\n      3063  0CF101A7   00000004    8        68\t00\t97\tCC\t00\t16\t39\tB3\r\n      3062  1FFFFFFF   00000004    8        00\t20\tFF\tFF\tFF\tFF\tFF\tFF\r\n      3052  1FFFFFFF   00000004    8        00\t20\tFF\tFF\tFF\tFF\tFF\tFF\r\n      3047  1FFFFFFF   00000004    8        00\t20\tFF\tFF\tFF\tFF\tFF\tFF\r\n      3046  18F121F0   00000004    8        09\t33\t00\t00\tFF\tFF\tB0\t01\r\n      3045  18F106A7   00000004    8        00\tF7\tFF\tFF\tFF\tFF\tFF\tAD\r\n      3045  0CF104A7   00000004    8        F0\t60\t22\tFC\tFF\tFF\tFF\t56\r\n      3044  0CF103A7   00000004    8        17\t1F\t08\t60\tB1\t1F\t08\t56\r\n      3083  0CF101A7   00000004    8        68\t00\t97\tCC\t00\t16\t39\tB4\r\n      3082  1FFFFFFF   00000004    8        00\t20\tFF\tFF\tFF\tFF\tFF\tFF\r\n      3072  1FFFFFFF   00000004    8        00\t20\tFF\tFF\tFF\tFF\tFF\tFF\r\n      3063  0CF102A7   00000004    8        30\t75\tE0\t2E\t80\tFF\tFF\tFD\r\n      3063  0CF101A7   00000004    8        68\t00\t97\tCC\t00\t16\t39\tB3\r\n      3062  1FFFFFFF   00000004    8        00\t20\tFF\tFF\tFF\tFF\tFF\tFF\r\n      3052  1FFFFFFF   00000004    8        00\t20\tFF\tFF\tFF\tFF\tFF\tFF\r\n      3047  1FFFFFFF   00000004    8        00\t20\tFF\tFF\tFF\tFF\tFF\tFF\r\n      3046  18F121F0   00000004    8        09\t33\t00\t00\tFF\tFF\tB0\t01\r\n      3045  18F106A7   00000004    8        00\tF7\tFF\tFF\tFF\tFF\tFF\tAD\r\n      3045  0CF104A7   00000004    8        F0\t60\t22\tFC\tFF\tFF\tFF\t56\r\n      3083  0CF102A7   00000004    8        30\t75\tE0\t2E\t80\tFF\tFF\tFD\r\n      3083  0CF101A7   00000004    8        68\t00\t97\tCC\t00\t16\t39\tB4\r\n      3082  1FFFFFFF   00000004    8        00\t20\tFF\tFF\tFF\tFF\tFF\tFF\r\n      3072  1FFFFFFF   00000004    8        00\t20\tFF\tFF\tFF\tFF\tFF\tFF\r\n      3063  0CF102A7   00000004    8        30\t75\tE0\t2E\t80\tFF\tFF\tFD\r\n      3063  0CF101A7   00000004    8        68\t00\t97\tCC\t00\t16\t39\tB3\r\n      3062  1FFFFFFF   00000004    8        00\t20\tFF\tFF\tFF\tFF\tFF\tFF\r\n      3052  1FFFFFFF   00000004    8        00\t20\tFF\tFF\tFF\tFF\tFF\tFF\r\n      3047  1FFFFFFF   00000004    8        00\t20\tFF\tFF\tFF\tFF\tFF\tFF\r\n      3046  18F121F0   00000004    8        09\t33\t00\t00\tFF\tFF\tB0\t01\r\n      3045  18F106A7   00000004    8        00\tF7\tFF\tFF\tFF\tFF\tFF\tAD\r\n      3092  1FFFFFFF   00000004    8        00\t20\tFF\tFF\tFF\tFF\tFF\tFF\r\n      3083  0CF102A7   00000004    8        30\t75\tE0\t2E\t80\tFF\tFF\tFD\r\n      3083  0CF101A7   00000004    8        68\t00\t97\tCC\t00\t16\t39\tB4\r\n      3082  1FFFFFFF   00000004    8        00\t20\tFF\tFF\tFF\tFF\tFF\tFF\r\n      3072  1FFFFFFF   00000004    8        00\t20\tFF\tFF\tFF\tFF\tFF\tFF\r\n      3063  0CF102A7   00000004    8        30\t75\tE0\t2E\t80\tFF\tFF\tFD\r\n      3063  0CF101A7   00000004    8        68\t00\t97\tCC\t00\t16\t39\tB3\r\n      3062  1FFFFFFF   00000004    8        00\t20\tFF\tFF\tFF\tFF\tFF\tFF\r\n      3052  1FFFFFFF   00000004    8        00\t20\tFF\tFF\tFF\tFF\tFF\tFF\r\n      3047  1FFFFFFF   00000004    8        00\t20\tFF\tFF\tFF\tFF\tFF\tFF\r\n      3046  18F121F0   00000004    8        09\t33\t00\t00\tFF\tFF\tB0\t01\r\n      3093  18F106A7   00000004    8        00\tF7\tFF\tFF\tFF\tFF\tFF\tAE\r\n      3092  1FFFFFFF   00000004    8        00\t20\tFF\tFF\tFF\tFF\tFF\tFF\r\n      3083  0CF102A7   00000004    8        30\t75\tE0\t2E\t80\tFF\tFF\tFD\r\n      3083  0CF101A7   00000004    8        68\t00\t97\tCC\t00\t16\t39\tB4\r\n      3082  1FFFFFFF   00000004    8        00\t20\tFF\tFF\tFF\tFF\tFF\tFF\r\n      3072  1FFFFFFF   00000004    8        00\t20\tFF\tFF\tFF\tFF\tFF\tFF\r\n      3063  0CF102A7   00000004    8        30\t75\tE0\t2E\t80\tFF\tFF\tFD\r\n      3063  0CF101A7   00000004    8        68\t00\t97\tCC\t00\t16\t39\tB3\r\n      3062  1FFFFFFF   00000004    8        00\t20\tFF\tFF\tFF\tFF\tFF\tFF\r\n      3052  1FFFFFFF   00000004    8        00\t20\tFF\tFF\tFF\tFF\tFF\tFF\r\n      3047  1FFFFFFF   00000004    8        00\t20\tFF\tFF\tFF\tFF\tFF\tFF\r\n      3102  1FFFFFFF   00000004    8        00\t00\tFF\tFF\tFF\tFF\tFF\tFF\r\n      3093  18F106A7   00000004    8        00\tF7\tFF\tFF\tFF\tFF\tFF\tAE\r\n      3092  1FFFFFFF   00000004    8        00\t20\tFF\tFF\tFF\tFF\tFF\tFF\r\n      3083  0CF102A7   00000004    8        30\t75\tE0\t2E\t80\tFF\tFF\tFD\r\n      3083  0CF101A7   00000004    8        68\t00\t97\tCC\t00\t16\t39\tB4\r\n      3082  1FFFFFFF   00000004    8        00\t20\tFF\tFF\tFF\tFF\tFF\tFF\r\n      3072  1FFFFFFF   00000004    8        00\t20\tFF\tFF\tFF\tFF\tFF\tFF\r\n      3063  0CF102A7   00000004    8        30\t75\tE0\t2E\t80\tFF\tFF\tFD\r\n      3063  0CF101A7   00000004    8        68\t00\t97\tCC\t00\t16\t39\tB3\r\n      3062  1FFFFFFF   00000004    8        00\t20\tFF\tFF\tFF\tFF\tFF\tFF\r\n      3052  1FFFFFFF   00000004    8        00\t20\tFF\tFF\tFF\tFF\tFF\tFF\r\n      3103  0CF101A7   00000004    8        68\t00\t97\tCC\t00\t16\t39\tB5\r\n      3102  1FFFFFFF   00000004    8        00\t00\tFF\tFF\tFF\tFF\tFF\tFF\r\n      3093  18F106A7   00000004    8        00\tF7\tFF\tFF\tFF\tFF\tFF\tAE\r\n      3092  1FFFFFFF   00000004    8        00\t20\tFF\tFF\tFF\tFF\tFF\tFF\r\n      3083  0CF102A7   00000004    8        30\t75\tE0\t2E\t80\tFF\tFF\tFD\r\n      3083  0CF101A7   00000004    8        68\t00\t97\tCC\t00\t16\t39\tB4\r\n      3082  1FFFFFFF   00000004    8        00\t20\tFF\tFF\tFF\tFF\tFF\tFF\r\n      3072  1FFFFFFF   00000004    8        00\t20\tFF\tFF\tFF\tFF\tFF\tFF\r\n      3063  0CF102A7   00000004    8        30\t75\tE0\t2E\t80\tFF\tFF\tFD\r\n      3063  0CF101A7   00000004    8        68\t00\t97\tCC\t00\t16\t39\tB3\r\n      3062  1FFFFFFF   00000004    8        00\t20\tFF\tFF\tFF\tFF\tFF\tFF\r\n      3103  0CF102A7   00000004    8        30\t75\tE0\t2E\t80\tFF\tFF\tFD\r\n      3103  0CF101A7   00000004    8        68\t00\t97\tCC\t00\t16\t39\tB5\r\n      3102  1FFFFFFF   00000004    8        00\t00\tFF\tFF\tFF\tFF\tFF\tFF\r\n      3093  18F106A7   00000004    8        00\tF7\tFF\tFF\tFF\tFF\tFF\tAE\r\n      3092  1FFFFFFF   00000004    8        00\t20\tFF\tFF\tFF\tFF\tFF\tFF\r\n      3083  0CF102A7   00000004    8        30\t75\tE0\t2E\t80\tFF\tFF\tFD\r\n      3083  0CF101A7   00000004    8        68\t00\t97\tCC\t00\t16\t39\tB4\r\n      3082  1FFFFFFF   00000004    8        00\t20\tFF\tFF\tFF\tFF\tFF\tFF\r\n      3072  1FFFFFFF   00000004    8        00\t20\tFF\tFF\tFF\tFF\tFF\tFF\r\n      3063  0CF102A7   00000004    8        30\t75\tE0\t2E\t80\tFF\tFF\tFD\r\n      3063  0CF101A7   00000004    8        68\t00\t97\tCC\t00\t16\t39\tB3\r\n      3112  1FFFFFFF   00000004    8        00\t20\tFF\tFF\tFF\tFF\tFF\tFF\r\n      3103  0CF102A7   00000004    8        30\t75\tE0\t2E\t80\tFF\tFF\tFD\r\n      3103  0CF101A7   00000004    8        68\t00\t97\tCC\t00\t16\t39\tB5\r\n      3102  1FFFFFFF   00000004    8        00\t00\tFF\tFF\tFF\tFF\tFF\tFF\r\n      3093  18F106A7   00000004    8        00\tF7\tFF\tFF\tFF\tFF\tFF\tAE\r\n      3092  1FFFFFFF   00000004    8        00\t20\tFF\tFF\tFF\tFF\tFF\tFF\r\n      3083  0CF102A7   00000004    8        30\t75\tE0\t2E\t80\tFF\tFF\tFD\r\n      3083  0CF101A7   00000004    8        68\t00\t97\tCC\t00\t16\t39\tB4\r\n      3082  1FFFFFFF   00000004    8        00\t20\tFF\tFF\tFF\tFF\tFF\tFF\r\n      3072  1FFFFFFF   00000004    8        00\t20\tFF\tFF\tFF\tFF\tFF\tFF\r\n      3063  0CF102A7   00000004    8        30\t75\tE0\t2E\t80\tFF\tFF\tFD\r\n      3122  1FFFFFFF   00000004    8        00\t00\tFF\tFF\tFF\tFF\tFF\tFF\r\n      3112  1FFFFFFF   00000004    8        00\t20\tFF\tFF\tFF\tFF\tFF\tFF\r\n      3103  0CF102A7   00000004    8        30\t75\tE0\t2E\t80\tFF\tFF\tFD\r\n      3103  0CF101A7   00000004    8        68\t00\t97\tCC\t00\t16\t39\tB5\r\n      3102  1FFFFFFF   00000004    8        00\t00\tFF\tFF\tFF\tFF\tFF\tFF\r\n      3093  18F106A7   00000004    8        00\tF7\tFF\tFF\tFF\tFF\tFF\tAE\r\n      3092  1FFFFFFF   00000004    8        00\t20\tFF\tFF\tFF\tFF\tFF\tFF\r\n      3083  0CF102A7   00000004    8        30\t75\tE0\t2E\t80\tFF\tFF\tFD\r\n      3083  0CF101A7 
